vi "ehl_init.vi"(8 "error in (no error)":errorcluster) -> (0 "error out":errorcluster, 2 "Event Registration Refnum":refnum<event-registration>, 3 "User Event out":refnum<user-event>)   [LabVIEW 2020]
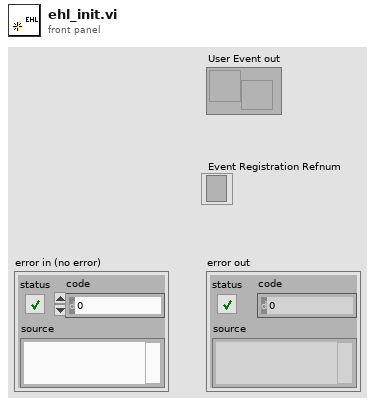
[diagram p1: front panel]
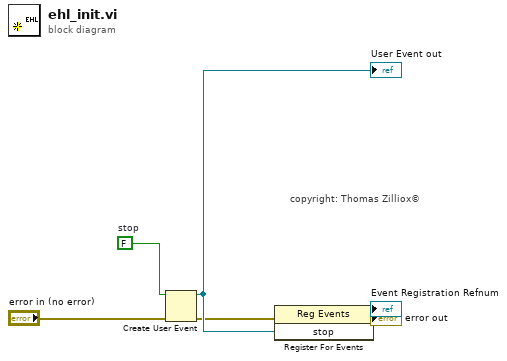
[diagram p0: block diagram]
diagram:
  w4 = FALSE  # stop
  # "copyright: Thomas Zilliox©"
  n1 = Create User Event(user event datatype=w4, error in="error in (no error)") -> (user event=w5:refnum<user-event>, error out=w3:errorcluster)
  "User Event out" <- w5
  n2 = register-events(error in=w3, w5) -> (reference out=→"Event Registration Refnum":refnum<event-registration>, error out=→"error out":errorcluster)  [unwired: 1 in]
